vi "read_params.vi"(8 "error in (no error)":errorcluster, 11 "MiniBatchDictionaryLearning in":refnum<class "MiniBatchDictionaryLearning.lvclass">) -> (0 "error out":errorcluster, 2 "params":T1={"n_components"={"n_components_type"="None", "n_components_int"=0.0}, "alpha"=1.0, "n_iter"=1000.0, "fit_algorithm"="lars", "n_jobs"=1.0, "batch_size"=3.0, "shuffle"=TRUE, "dict_init"=[], "transform_algorithm"="omp", "transform_n_nonzero_coefs"={"transform_n_nonzero_coefs_type"="None", "transform_n_nonzero_coefs_int"=0.0}, "transform_alpha"=1.0, "verbose"=FALSE, "split_sign"=FALSE, "random_state"=0.0, "positive_code"=FALSE, "positive_dict"=FALSE, "transform_max_iter"=1000.0}, 3 "MiniBatchDictionaryLearning out":refnum<class "MiniBatchDictionaryLearning.lvclass">)   [LabVIEW 2020, in "MiniBatchDictionaryLearning.lvclass"]
uses:
  MiniBatchDictionaryLearning.lvclass
  Controls/mini_batch_dictionary_learning_params.ctl
  MiniBatchDictionaryLearning.lvclass/MiniBatchDictionaryLearning.ctl
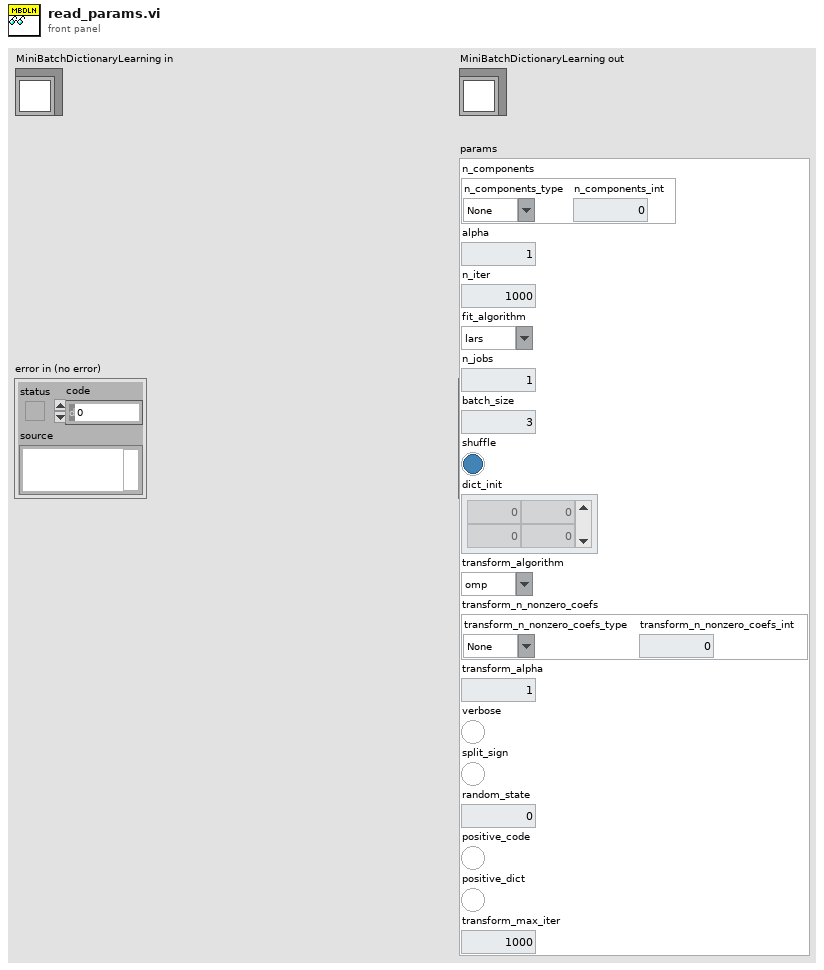
[diagram p1: front panel]
types:
  T1 = typedef "mini_batch_dictionary_learning_params.ctl" = cluster{"n_components":cluster{"n_components_type":string, "n_components_int":dbl}, "alpha":dbl, "n_iter":dbl, "fit_algorithm":string, "n_jobs":dbl, "batch_size":dbl, "shuffle":bool, "dict_init":dbl[][], "transform_algorithm":string, "transform_n_nonzero_coefs":cluster{"transform_n_nonzero_coefs_type":string, "transform_n_nonzero_coefs_int":dbl}, "transform_alpha":dbl, "verbose":bool, "split_sign":bool, "random_state":dbl, "positive_code":bool, "positive_dict":bool, "transform_max_iter":dbl}
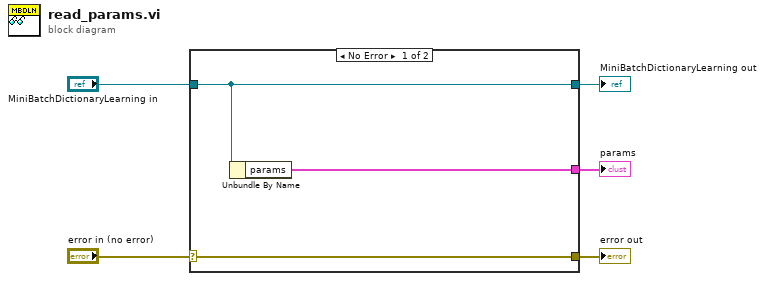
[diagram p0: block diagram]
diagram:
  n1 = case shown="No Error" "error in (no error)" {
    selector: "error in (no error)" -> [w8 w9]
    tunnel: [w8 w9] -> w4
    tunnel: [w7 w10] -> w2
    tunnel: "MiniBatchDictionaryLearning in" -> [w7 w10]
    tunnel: [w6 _] -> w1
    frame No Error {
      n2 = Unbundle By Name(w7) -> ("params"=w6:T1)
    }
    frame Error {
    }
  }
  "error out" <- w4
  "MiniBatchDictionaryLearning out" <- w2
  "params" <- w1
